vi "HP4284A Compensation Instruction.vi"(8 "error in (no error)":errorcluster, 11 "VISA resource name":refnum<visa-resource-name>) -> (0 "error out":errorcluster, 3 "VISA resource name out":refnum<visa-resource-name>)   [LabVIEW 2015, in "Agilent 428X Series.lvlib"]
uses:
  Agilent 428X Series.lvlib
panel:
  out "?":string="MEASUREMENT IN PROGRESS...\n            PLEASE WAIT..."
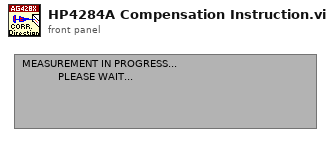
[diagram p1: front panel]
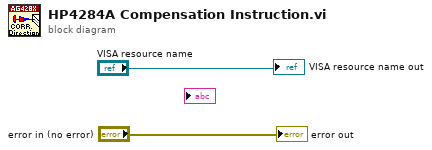
[diagram p0: block diagram]
diagram:
  "error out" <- "error in (no error)"
  "VISA resource name out" <- "VISA resource name"
